vi "run_profile.vi"(7 "queue":T2, 8 "error in (no error)":errorcluster, 10 "cycle":i32, 11 "profile":T1[](array[typedef])) -> (0 "error out":errorcluster)   [LabVIEW 2019]
uses:
  core_dataRefCluster.ctl
  core_dataRef.ctl
  core_dataCluster.ctl
  core_setup.ctl
  <vilib>/Platform/TimedLoop/XDataNode/timing_clust.ctl
  <vilib>/Platform/TimedLoop/XDataNode/nitl_modes.ctl
  <vilib>/Platform/TimedLoop/XDataNode/wakeup.ctl
  profile value.ctl
  <vilib>/Platform/TimedLoop/XDataNode/XDataNode.xnode
  <vilib>/Platform/TimedLoop/XDataNode/XDNodeRunTimeDep.lvlib
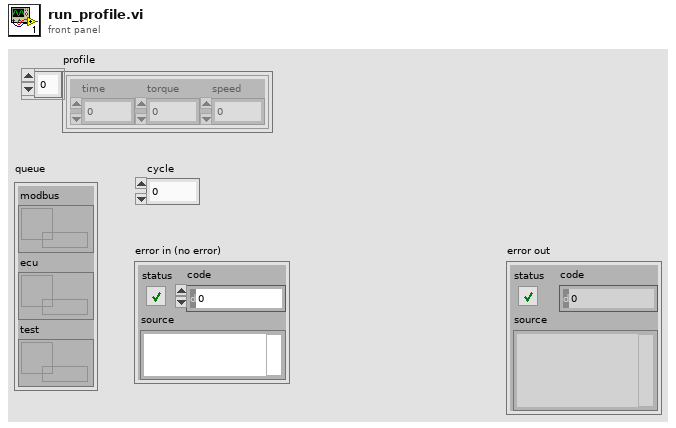
[diagram p1: front panel]
types:
  T1 = typedef "core_setup.ctl" = cluster{"time":i32, "torque":dbl, "speed":i32}
  T2 = typedef "core_dataRefCluster.ctl" = cluster{"modbus":T3, "ecu":T3, "test":T3}
  T3 = typedef "core_dataRef.ctl" = refnum<queue>
  T4 = typedef "core_dataCluster.ctl" = cluster{"cmd":string, "data":variant}
  T5 = typedef "profile value.ctl" = cluster{"time in":i32, "speed":dbl, "Torque":dbl}
  T6 = typedef "XDNodeRunTimeDep.lvlib/timing_clust.ctl" = cluster{"Expected End [f-1]":u64, "Actual End [f-1]":u64, "Finished Late? [f-1]":bool, "Expected End [i-1]":u64, "Actual End [i-1]":u64, "Finished Late? [i-1]":bool, "Expected Start [i]":u64, "Actual Start [i]":u64, "Expected Start [f]":u64, "Actual Start [f]":u64, "Source Name":string, "Structure Name":string, "Period":i64, "Deadline":i64, "Offset":i64, "Start":i64, "Priority":i32, "Timeout":i32, "Mode":T7, "Wakeup Reason":T8, "Error":errorcluster, "Source Type":string, "Secondary Source Type":string, "Global End Time":u64, "Global Start Time":u64, "Frame Duration":u64, "Iteration Duration":u64, "Assigned CPU":i32, "I/O Scan Engine Mode":u32}
  T7 = typedef "XDNodeRunTimeDep.lvlib/nitl_modes.ctl" = enum32{"No Change", "Process missed periods, maintain original phase", "Discard missed periods, maintain original phase", "Process missed periods, ignore original phase", "Discard missed periods, ignore original phase"}
  T8 = typedef "XDNodeRunTimeDep.lvlib/wakeup.ctl" = enum32{"Normal", "Aborted", "Asynchronous wakeup", "Timing source error", "Timed loop error", "Timeout"}
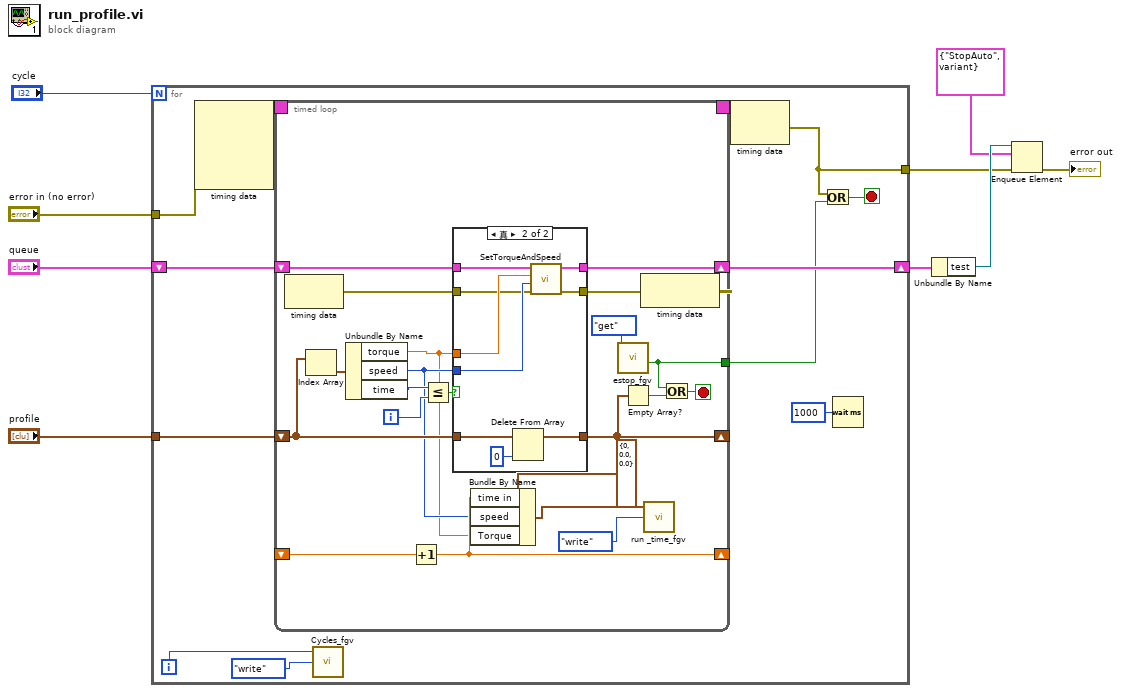
[diagram p0: block diagram]
diagram:
  n1 = for {
    N: "cycle" -> [_]
    tunnel: "profile" -> [w19]
    tunnel: "error in (no error)" -> [w17]
    tunnel: [w14] -> w1
    shift-right: [w16] -> w3
    shift-left: "queue" -> [w18]
    i -> [w10]
    stop <- w13 stop-if-true
    n2 = node-c288(w17) -> (w21:T6)  [unwired: 3 in]
    n3 = timed-loop {
      timing: w21 -> [_]
      timing-out: [_] -> w20
      shift-right: [w37] -> _
      shift-left: w19 -> [w38]
      shift-right: [w33] -> w16
      shift-left: w18 -> [w34]
      tunnel: [w29] -> w12
      shift-right: [w27] -> _
      shift-left: _ -> [w28]
      i -> [w40]
      stop <- w30 stop-if-true
      n4 = node-c288() -> (w35:errorcluster)  [unwired: 1 in]
      n5 = Index Array(array=w38) -> (element=w42:T1)  [unwired: 1 in]
      n6 = Unbundle By Name(w42) -> ("torque"=w25:dbl, "speed"=w26:i32, "time"=w41:i32)
      n7 = Increment(x=w28) -> (x+1=w27:dbl)
      n8 = Less Or Equal?(x=w41, y=w40) -> (x <= y?=w39:bool)
      n9 = case shown="真" w39 {
        tunnel: w38 -> [w45 w54]
        tunnel: [w45 w52] -> w37
        tunnel: [w44 w47] -> w36
        tunnel: w26 -> [_ w50]
        tunnel: w35 -> [w44 w48]
        tunnel: w34 -> [w43 w51]
        tunnel: w25 -> [_ w49]
        tunnel: [w43 w46] -> w33
        frame False {
        }
        frame True {
          n10 = Delete From Array(array=w54, index=0) -> (array with subset deleted=w52:T1[])  [unwired: 1 in, 1 out]
          n11 = call "SetTorqueAndSpeed.vi"("error in (no error)"=w48, "Speed"=w50, "Torque"=w49, "Cluster in"=w51) -> ("error out"=w47:errorcluster, "Cluster out"=w46:T2)  [unwired: 6 in]
        }
      }
      n12 = Bundle By Name(cluster=T5 {"time in"=0, "speed"=0.0, "Torque"=0.0} ("Value  in"), "time in"=w27, "speed"=w26, "Torque"=w25) -> (w22:T5)
      n13 = call "estop_fgv.vi"("Enum"=enum16{"set", "get"}."get") -> ("indicator"=w29:bool)  [unwired: 9 in, 1 out]
      n14 = Empty Array?(array=w37) -> (empty?=w31:bool)
      n15 = node-c288(w36) -> ()  [unwired: 1 out]
      n16 = call "run _time_fgv .vi"("mode"=enum16{"read", "write"}."write", "Value  in"=w22) -> ()  [unwired: 1 in, 2 out]
      n17 = Or(x=w29, y=w31) -> (x .or. y?=w30:bool)
    }
    n18 = call "Cycles_fgv.vi"("mode"=enum16{"read", "write"}."write", "IN"=w10) -> ()  [unwired: 1 in, 2 out]
    n19 = node-c288(w20) -> (w14:errorcluster)
    n20 = Or(x=w14, y=w12) -> (x .or. y?=w13:bool)
    n21 = Wait (ms)(milliseconds to wait=u32 1000) -> ()  [unwired: 1 out]
  }
  n22 = Unbundle By Name(w3) -> ("test"=w5:T3)
  n23 = Enqueue Element(queue=w5, element=T4 {"cmd"="StopAuto", "data"=variant}, error in (no error)=w1) -> (error out=→"error out":errorcluster)  [unwired: 1 in, 2 out]
